vi "PhotonPipelineResult_GetBestTarget.vi"(11 "PhotonPipelineResult":T6 {"Targets"."CameraToTarget"."ROTATION"."SIN" format="%13.4f"; "Targets"."CameraToTarget"."ROTATION"."COS" format="%13.4f"; "Targets"."CameraToTarget"."ROTATION"."VALUE" format="%13.4f"; "Targets"."CameraToTarget"."TRANSLATION"."Y" format="%14.3f"; "Targets"."CameraToTarget"."TRANSLATION"."X" format="%14.3f"}) -> (3 "PhotonTrackedTarget":T1={"Yaw"=0.0, "Pitch"=0.0, "Area"=0.0, "Skew"=0.0, "TargetCorners"=[], "CameraToTarget"={"TRANSLATION"={"X"=0.0, "Y"=0.0}, "ROTATION"={"VALUE"=0.0, "COS"=1.0, "SIN"=0.0}}, "FiducialId"=0} {"CameraToTarget"."ROTATION"."SIN" format="%13.4f"; "CameraToTarget"."ROTATION"."COS" format="%13.4f"; "CameraToTarget"."ROTATION"."VALUE" format="%13.4f"; "CameraToTarget"."TRANSLATION"."Y" format="%14.3f"; "CameraToTarget"."TRANSLATION"."X" format="%14.3f"})   [LabVIEW 2020, in "PhotonVisionLib.lvlib"]
doc: "Returns the best target in this pipeline result. If there are no targets, this method will return an empty target. The best target is determined by the target sort mode in the PhotonVision UI.\n\nInputs:\n - PipelineResult -- Parsed PipelineResult cluster.\n\nOutputs:\n - TrackedTarget -- Cluster containing the best target"
uses:
  PhotonVisionLib.lvlib
  TypeDef/PhotonPipelineResultType.ctl
  TypeDef/PhotonTrackedTargetType.ctl
  TypeDef/TargetCornerType.ctl
  <vilib>/Rock Robotics/WPI/ThirdParty/JAS_Junk/TrajLib/TRANSFORM2D.ctl
  <vilib>/Rock Robotics/WPI/ThirdParty/JAS_Junk/TrajLib/TRANSLATION2D.ctl
  <vilib>/Rock Robotics/WPI/ThirdParty/JAS_Junk/TrajLib/ROTATION2D.ctl
  <vilib>/Rock Robotics/WPI/ThirdParty/JAS_Junk/TrajLib/Trajectory_Library.lvlib
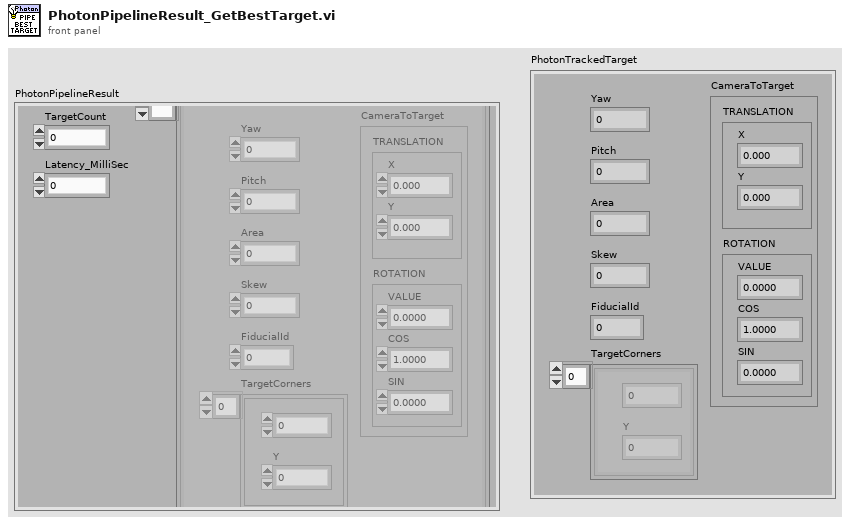
[diagram p1: front panel]
types:
  T1 = typedef "PhotonVisionLib.lvlib/PhotonTrackedTargetType.ctl" = cluster{"Yaw":dbl, "Pitch":dbl, "Area":dbl, "Skew":dbl, "TargetCorners":T2[], "CameraToTarget":T3, "FiducialId":i32}
  T2 = typedef "PhotonVisionLib.lvlib/TargetCornerType.ctl" = cluster{"X":dbl, "Y":dbl}
  T3 = typedef "Trajectory_Library.lvlib/TRANSFORM2D.ctl" = cluster{"TRANSLATION":T4, "ROTATION":T5}
  T4 = typedef "Trajectory_Library.lvlib/TRANSLATION2D.ctl" = cluster{"X":dbl, "Y":dbl}
  T5 = typedef "Trajectory_Library.lvlib/ROTATION2D.ctl" = cluster{"VALUE":dbl, "COS":dbl, "SIN":dbl}
  T6 = typedef "PhotonVisionLib.lvlib/PhotonPipelineResultType.ctl" = cluster{"TargetCount":i32, "Latency_MilliSec":dbl, "Targets":T1[]}
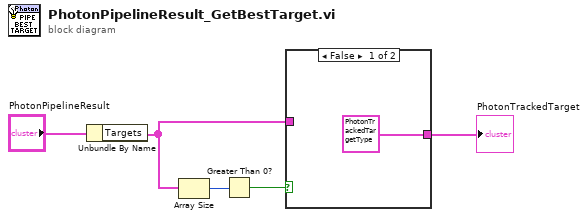
[diagram p0: block diagram]
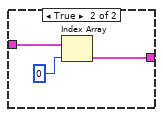
[diagram p2: hidden frame]
diagram:
  n1 = Unbundle By Name("PhotonPipelineResult") -> ("Targets"=w2:T1[])
  n2 = Array Size(array=w2) -> (size(s)=w4:i32)
  n3 = Greater Than 0?(x=w4) -> (x > 0?=w3:bool)
  n4 = case shown="False" w3 {
    tunnel: w2 -> [_ w8]
    tunnel: [T1 {"Yaw"=0.0, "Pitch"=0.0, "Area"=0.0, "Skew"=0.0, "TargetCorners"=[], "CameraToTarget"={"TRANSLATION"={"X"=0.0, "Y"=0.0}, "ROTATION"={"VALUE"=0.0, "COS"=1.0, "SIN"=0.0}}, "FiducialId"=0} ("PhotonTrackedTarget") w7] -> w1
    frame False {
    }
    frame True {
      n5 = Index Array(array=w8, index=0) -> (element=w7:T1)
    }
  }
  "PhotonTrackedTarget" <- w1
